vi "niFPGA FFT Calculate Addresses.vi"(0 "butterfly count":u16, 5 "current stage":u8, 7 "K - 1":u8=3, 9 "K - 17":i8=3) -> (4 "switch?":bool, 6 "address":u16, 8 "twiddle index":u16)   [LabVIEW 2017]
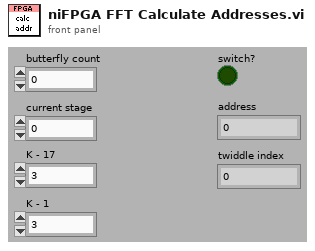
[diagram p1: front panel]
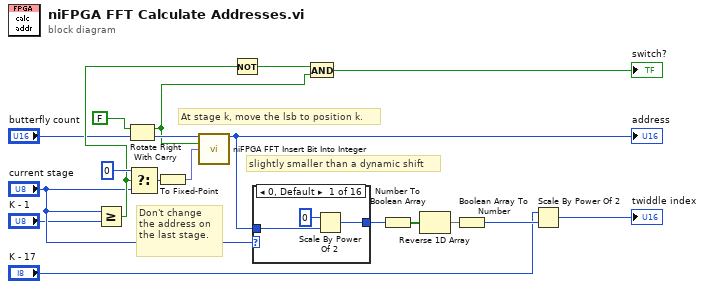
[diagram p0: block diagram]
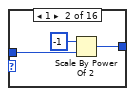
[diagram p2: hidden frame]
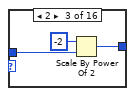
[diagram p3: hidden frame]
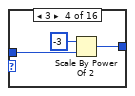
[diagram p4: hidden frame]
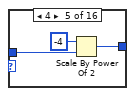
[diagram p5: hidden frame]
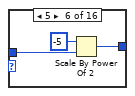
[diagram p6: hidden frame]
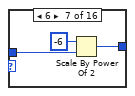
[diagram p7: hidden frame]
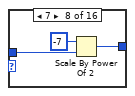
[diagram p8: hidden frame]
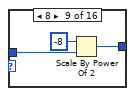
[diagram p9: hidden frame]
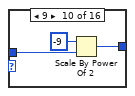
[diagram p10: hidden frame]
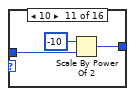
[diagram p11: hidden frame]
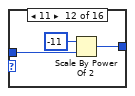
[diagram p12: hidden frame]
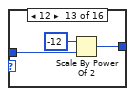
[diagram p13: hidden frame]
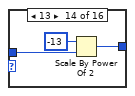
[diagram p14: hidden frame]
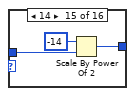
[diagram p15: hidden frame]
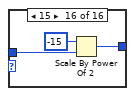
[diagram p16: hidden frame]
diagram:
  # "At stage k, move the lsb to position k."
  # "Don't change the address on the last stage."
  # "slightly smaller than a dynamic shift"
  n1 = Greater Or Equal?(x="current stage", y="K - 1") -> (x >= y?=w12:bool)
  n2 = Rotate Right With Carry(2:"butterfly count", 3:FALSE ("carry")) -> (0:w16:u16, 1:w14:bool)
  n3 = Select(t=u8 0, s=w12, f="current stage") -> (s? t:f=w18:u8)
  n4 = To Fixed-Point(number=w18) -> (fixed-point=w17:fxp<+,4,4>)  [unwired: 1 out]
  n5 = call <vilib>:"niFPGA FFT Insert Bit Into Integer.vi"("integer"=w16, "input value"=w14, "index"=w17) -> ("output integer"=w9:u16)  [unwired: 12 out]
  "address" <- w9
  n6 = Not(x=w12) -> (.not. x?=w11:bool)
  n7 = case shown="0, Default" "current stage" {
    tunnel: w9 -> [w22 w23 w26 w29 w32 w37 w40 w43 w46 w49 w52 w55 w58 w61 w64 w67]
    tunnel: [w20 w24 w27 w30 w33 w35 w38 w41 w44 w47 w50 w53 w56 w59 w62 w65] -> w6
    frame 0, Default {
      n8 = Scale By Power Of 2(n=0, x=w22) -> (x*2^n=w20:u16)
    }
    frame 1 {
      n9 = Scale By Power Of 2(n=-1, x=w23) -> (x*2^n=w24:u16)
    }
    frame 2 {
      n10 = Scale By Power Of 2(n=-2, x=w26) -> (x*2^n=w27:u16)
    }
    frame 3 {
      n11 = Scale By Power Of 2(n=-3, x=w29) -> (x*2^n=w30:u16)
    }
    frame 4 {
      n12 = Scale By Power Of 2(n=-4, x=w32) -> (x*2^n=w33:u16)
    }
    frame 5 {
      n13 = Scale By Power Of 2(n=-5, x=w37) -> (x*2^n=w35:u16)
    }
    frame 6 {
      n14 = Scale By Power Of 2(n=-6, x=w40) -> (x*2^n=w38:u16)
    }
    frame 7 {
      n15 = Scale By Power Of 2(n=-7, x=w43) -> (x*2^n=w41:u16)
    }
    frame 8 {
      n16 = Scale By Power Of 2(n=-8, x=w46) -> (x*2^n=w44:u16)
    }
    frame 9 {
      n17 = Scale By Power Of 2(n=-9, x=w49) -> (x*2^n=w47:u16)
    }
    frame 10 {
      n18 = Scale By Power Of 2(n=-10, x=w52) -> (x*2^n=w50:u16)
    }
    frame 11 {
      n19 = Scale By Power Of 2(n=-11, x=w55) -> (x*2^n=w53:u16)
    }
    frame 12 {
      n20 = Scale By Power Of 2(n=-12, x=w58) -> (x*2^n=w56:u16)
    }
    frame 13 {
      n21 = Scale By Power Of 2(n=-13, x=w61) -> (x*2^n=w59:u16)
    }
    frame 14 {
      n22 = Scale By Power Of 2(n=-14, x=w64) -> (x*2^n=w62:u16)
    }
    frame 15 {
      n23 = Scale By Power Of 2(n=-15, x=w67) -> (x*2^n=w65:u16)
    }
  }
  n24 = And(x=w11, y=w14) -> (x .and. y?=→"switch?":bool)
  n25 = Number To Boolean Array(number=w6) -> (Boolean array=w7:bool[])
  n26 = Reverse 1D Array(array=w7) -> (reversed array=w5:bool[])
  n27 = Boolean Array To Number(Boolean array=w5) -> (number=w4:u16)
  n28 = Scale By Power Of 2(n="K - 17", x=w4) -> (x*2^n=→"twiddle index":u16)
